vi "Open Report.vi"(0 "reference in":refnum<class "Reporter.lvclass">, 5 "error in (no error)":errorcluster) -> (14 "reference out":refnum<class "Reporter.lvclass">, 19 "error out":errorcluster)   [LabVIEW 2020, in "Reporter.lvclass"]
uses:
  Reporter.lvclass
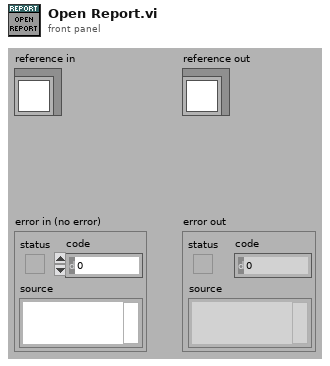
[diagram p1: front panel]
types:
  T1 = enum16{"open", "replace", "create", "open or create", "replace or create", "replace or create with confirmation"}
  T2 = typedef "Reporter.lvclass/ObjectAttributes.ctl" = cluster{"LCR":refnum<class "BKP-891 LCR Meter.lvclass">, "PSU":refnum<class "BKP-911x Power Supply.lvclass">, "NI-DAQmx":refnum<class "NI-DAQmx.lvclass">, "Signal List":T3[], "Latest Values":dbl[], "All Latest Values":dbl[], "All Signal List":T3[], "Report Directory":path, "Report File Ref":refnum<file>}
  T3 = typedef "IO Signal List.ctl" = enum16{"Timestamp", "PSU_FB_U_VDC", "PSU_FB_I_AMP", "PSU_FB_W_WATT", "PSU_CMD_U_VDC", "PSU_CMD_I_AMP", "PSU_CMD_OUTPUT", "LCR_PRIMARY", "LCR_SECONDARY", "UV_R_Ohm", "UW_R_Ohm", "VW_R_Ohm", "UV_L_H", "UW_L_H", "VW_L_H", "U_U_VDC", "V_U_VDC", "W_U_VDC", "U_I_AMP", "V_I_AMP", "W_I_AMP", "PWM_CMD_DC_%", "PWM_CMD_VDC", "PWM_CMD_Hz", "PWM_FB_DC_%", "PWM_FB_VDC", "PWM_FB_Hz", "DO_RELAY_U_LCR_A", "DO_RELAY_V_LCR_A", "DO_RELAY_V_LCR_B", "DO_RELAY_W_LCR_B", "DIFF_UV_UW_L_H", "DIFF_UV_VW_L_H", "DIFF_UW_VW_L_H", "DIFF_UV_UW_R_Ohm", "DIFF_UV_VW_R_Ohm", "DIFF_UW_VW_R_Ohm", "DIFF_UV_U_VDC", "DIFF_UW_U_VDC", "DIFF_VW_U_VDC"}
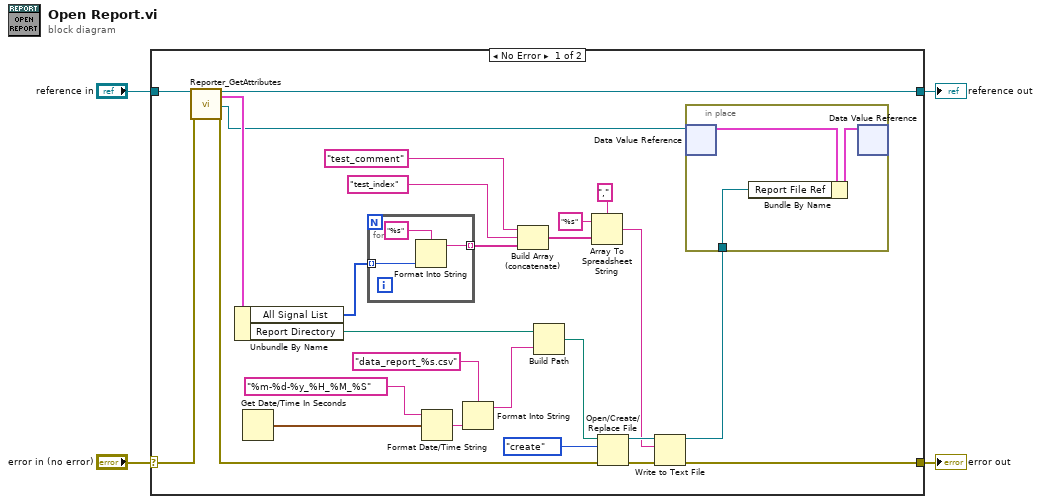
[diagram p0: block diagram]
diagram:
  n1 = case shown="No Error" "error in (no error)" {
    selector: "error in (no error)" -> [w30 w38]
    tunnel: [w13 w38] -> w3
    tunnel: [w27 w37] -> w1
    tunnel: "reference in" -> [w28 w37]
    frame No Error {
      n2 = call "Reporter_GetAttributes.vi"("reference in"=w28, "error in (no error)"=w30) -> ("reference out"=w27:refnum<class "Reporter.lvclass">, "Data"=w29:T2, "DataRef"=w19:refnum<data-value>, "error out"=w24:errorcluster)  [unwired: 14 in]
      n3 = Unbundle By Name(w29) -> ("All Signal List"=w12:T3[], "Report Directory"=w26:path)
      n4 = Get Date/Time In Seconds() -> (seconds since 1Jan1904=w25:timestamp)
      n5 = for {
        tunnel: w12 -> [w33] mode=indexing
        tunnel: [w31] -> w8 mode=indexing
        n6 = Format Into String(format string="%s", w33) -> (resulting string=w31:string)  [unwired: 2 in, 1 out]
      }
      n7 = Format Date/Time String(time format string (%c)="%m-%d-%y_%H_%M_%S", seconds (now)=w25) -> (date/time string=w21:string)  [unwired: 1 in]
      n8 = Format Into String(format string="data_report_%s.csv", w21) -> (resulting string=w20:string)  [unwired: 2 in, 1 out]
      n9 = Build Array (concatenate)("test_comment" ("format string"), "test_index" ("format string"), w8) -> (w7:string[])
      n10 = Build Path(base path=w26, name or relative path=w20) -> (appended path=w23:path)
      n11 = Array To Spreadsheet String(delimiter (Tab)=",", array=w7, 3:"%s" ("format string")) -> (spreadsheet string=w9:string)
      n12 = Open/Create/Replace File(file path (use dialog)=w23, error in=w24, operation (0:open)=T1."create") -> (refnum out=w15:refnum<file>, error out=w16:errorcluster)  [unwired: 3 in, 1 out]
      n13 = Write to Text File(file (use dialog)=w15, text=w9, error in=w16) -> (refnum out=w14:refnum<file>, error out=w13:errorcluster)  [unwired: 1 in, 1 out]
      n14 = in-place {
        in-place-border: w14 -> [w34]
        n15 = in-place-dvr #1(w19) -> (w36:T2)  [unwired: 1 out]
        n16 = Bundle By Name(cluster=w36, "Report File Ref"=w34) -> (w35:T2)
        n17 = in-place-dvr #1(w35) -> ()  [unwired: 2 out]
      }
    }
    frame Error {
    }
  }
  "error out" <- w3
  "reference out" <- w1
